vi "init.vi"(8 "error in (no error)":errorcluster, 11 "IDE simple in":refnum<class "LF2R IDE.lvclass">) -> (0 "error out":errorcluster, 3 "IDE simple out":refnum<class "LF2R IDE.lvclass">)   [LabVIEW 2018, in "LF2R IDE.lvlib" / "LF2R IDE.lvclass"]
uses:
  LF2R IDE.lvclass
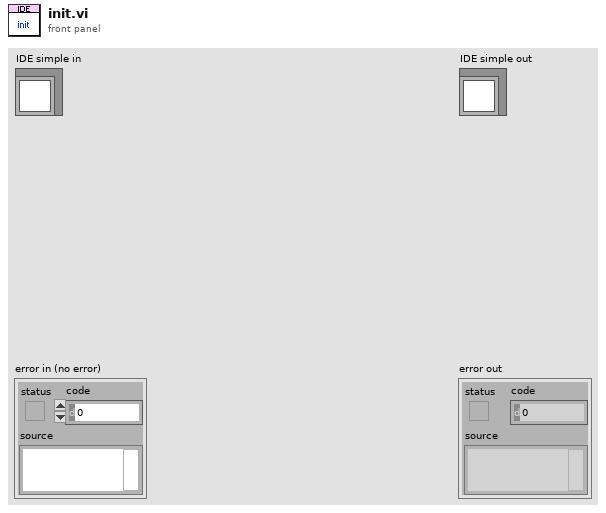
[diagram p1: front panel]
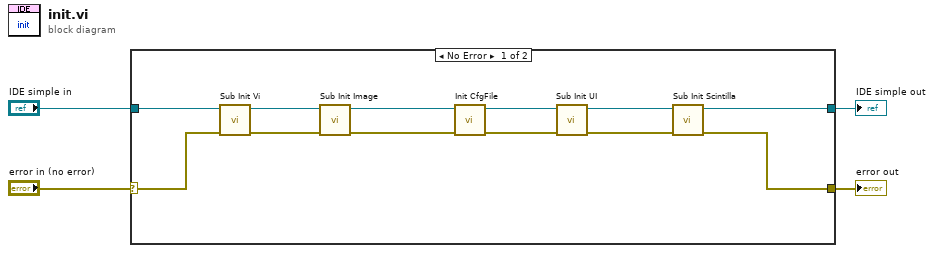
[diagram p0: block diagram]
diagram:
  n1 = case shown="No Error" "error in (no error)" {
    selector: "error in (no error)" -> [w15 w18]
    tunnel: [w13 w18] -> w3
    tunnel: [w14 w17] -> w1
    tunnel: "IDE simple in" -> [w16 w17]
    frame No Error {
      n2 = call "Sub Init Vi.vi"("error in (no error)"=w15, "IDE simple in"=w16) -> ("error out"=w11:errorcluster, "IDE simple out"=w12:refnum<class "LF2R IDE.lvclass">)  [unwired: 8 in]
      n3 = call "Sub Init Image.vi"("error in (no error)"=w11, "LF2R IDE in"=w12) -> ("error out"=w9:errorcluster, "LF2R IDE out"=w10:refnum<class "LF2R IDE.lvclass">)  [unwired: 8 in]
      n4 = call "Init CfgFile.vi"("error in (no error)"=w9, "LF2R IDE in"=w10) -> ("error out"=w7:errorcluster, "LF2R IDE out"=w8:refnum<class "LF2R IDE.lvclass">)  [unwired: 8 in]
      n5 = call "Sub Init UI.vi"("error in (no error)"=w7, "LF2R IDE in"=w8) -> ("error out"=w5:errorcluster, "LF2R IDE out"=w6:refnum<class "LF2R IDE.lvclass">)  [unwired: 8 in]
      n6 = call "Sub Init Scintilla.vi"("error in (no error)"=w5, "LF2R IDE in"=w6) -> ("error out"=w13:errorcluster, "LF2R IDE out"=w14:refnum<class "LF2R IDE.lvclass">)  [unwired: 8 in]
    }
    frame Error {
    }
  }
  "error out" <- w3
  "IDE simple out" <- w1
